vi "Configure Step.vi"(0 "VISA resource name":refnum<visa-resource-name>, 1 "Output AC Voltage Frequency (60  Hz)":dbl=60.0 min=45.0 max=1000.0 format="%.1p", 2 "Output AC Voltage (115 V)":dbl=115.0 min=0.0 max=300.0 format="%.1f", 3 "Step Prompt":T1={"Enable Prompt"=FALSE, "Prompt ( )"=" "}, 5 "Step (1)":i32=1 min=1 max=9 step=1, 7 "Step Cycle (1)":i32=1 min=0 max=9999 step=1, 9 "Enable Step Connection (F:Disable)":bool, 11 "error in (no error)":errorcluster, 12 "Voltage Range Mode (1:Auto)":u16(ring)=1 items=["High", "Auto"], 13 "Start Angle (0)":i32 min=0 max=359, 14 "End Angle: (0)":i32 min=0 max=359) -> (4 "VISA resource name out":refnum<visa-resource-name>, 15 "error out":errorcluster)   [LabVIEW 2016, in "APT 300XAC Series.lvlib"]
doc: "Configures the user specified step and its parameters in the current Memory location (Use \"Configure Memory.vi\" to select the desired memory)\n\nNote : Run \"Configure Program Mode.vi\" to make sure the instrument is in <B>Program Mode</B> before using this VI"
uses:
  APT 300XAC Series.lvlib
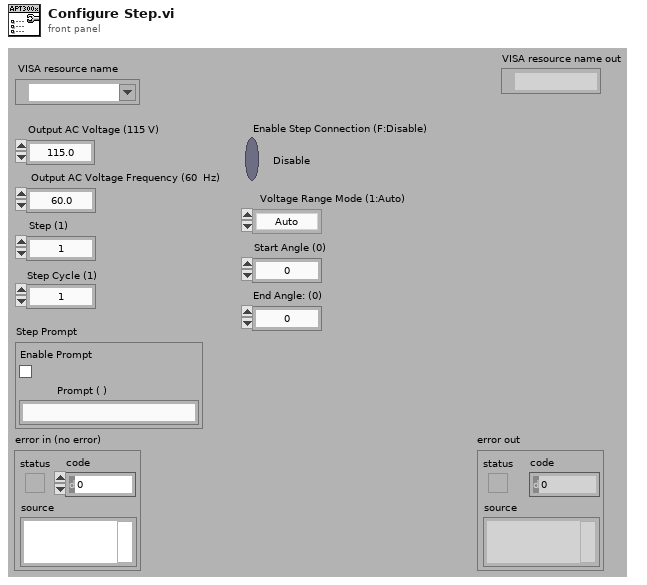
[diagram p1: front panel]
types:
  T1 = cluster{"Enable Prompt":bool, "Prompt ( )":string}
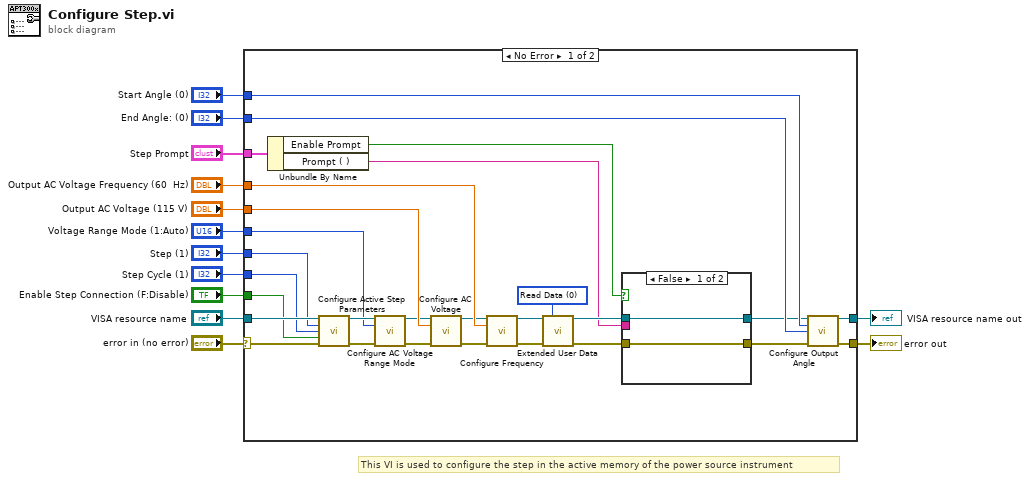
[diagram p0: block diagram]
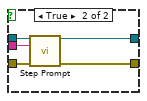
[diagram p2: hidden frame]
diagram:
  # "This VI is used to configure the step in the active memory of the power source instrument"
  n1 = case shown="No Error" "error in (no error)" {
    selector: "error in (no error)" -> [w40 w50]
    tunnel: [w27 w50] -> w13
    tunnel: [w28 w49] -> w12
    tunnel: "VISA resource name" -> [w41 w49]
    tunnel: "Output AC Voltage Frequency (60  Hz)" -> [w39 _]
    tunnel: "Step Cycle (1)" -> [w38 _]
    tunnel: "Enable Step Connection (F:Disable)" -> [w37 _]
    tunnel: "Step (1)" -> [w36 _]
    tunnel: "Output AC Voltage (115 V)" -> [w30 _]
    tunnel: "Voltage Range Mode (1:Auto)" -> [w29 _]
    tunnel: "Start Angle (0)" -> [w23 _]
    tunnel: "End Angle: (0)" -> [w22 _]
    tunnel: "Step Prompt" -> [w17 _]
    frame No Error {
      w24 = u16 0 items=["Read Data", "Write Data", "Clear Data", "Clear ALL Data"] ("Action")
      n2 = Unbundle By Name(w17) -> ("Enable Prompt"=w15:bool, "Prompt ( )"=w16:string)
      n3 = call "Configure Active Step Parameters.vi"("VISA resource name"=w41, "Step (1)"=w36, "Step Cycle (1)"=w38, "Enable Step Connection (F:Disable)"=w37, "error in (no error)"=w40) -> ("VISA resource name out"=w35:refnum<visa-resource-name>, "error out"=w34:errorcluster)  [unwired: 9 in]
      n4 = call "Configure AC Voltage Range Mode.vi"("VISA resource name"=w35, "Voltage Range Mode (1:Auto)"=w29, "error in (no error)"=w34) -> ("VISA resource name out"=w14:refnum<visa-resource-name>, "error out"=w33:errorcluster)  [unwired: 11 in]
      n5 = call "Configure AC Voltage.vi"("VISA resource name"=w14, "Output AC Voltage (115 V)"=w30, "error in (no error)"=w33) -> ("VISA resource name out"=w31:refnum<visa-resource-name>, "error out"=w32:errorcluster)  [unwired: 11 in]
      n6 = call "Configure Frequency.vi"("VISA resource name"=w31, "Output AC Voltage Frequency (60  Hz)"=w39, "error in (no error)"=w32) -> ("VISA resource name out"=w25:refnum<visa-resource-name>, "error out"=w26:errorcluster)  [unwired: 11 in]
      n7 = call "Extended User Data.vi"("VISA resource name"=w25, "Action"=w24, "Error In (no error)"=w26) -> ("VISA resource name out"=w21:refnum<visa-resource-name>, "Error Out"=w19:errorcluster)  [unwired: 10 in, 1 out]
      n8 = case shown="False" w15 {
        tunnel: w21 -> [w43 w48]
        tunnel: [w43 w47] -> w20
        tunnel: w19 -> [w42 w46]
        tunnel: [w42 w45] -> w18
        tunnel: w16 -> [_ w44]
        frame False {
        }
        frame True {
          n9 = call "Step Prompt.vi"("VISA resource name"=w48, "Prompt ( )"=w44, "error in (no error)"=w46) -> ("VISA resource name out"=w47:refnum<visa-resource-name>, "error out"=w45:errorcluster)  [unwired: 11 in]
        }
      }
      n10 = call "Configure Output Angle.vi"("VISA resource name"=w20, "Start Angle (0)"=w23, "End Angle: (0)"=w22, "error in (no error)"=w18) -> ("VISA resource name out"=w28:refnum<visa-resource-name>, "error out"=w27:errorcluster)  [unwired: 10 in]
    }
    frame Error {
    }
  }
  "error out" <- w13
  "VISA resource name out" <- w12
